vi "Measurement Coordinate Set.vi"(7 "CoordSys Type":T3(ring), 8 "error in (no error)":errorcluster, 9 "Angle (deg)":sgl, 10 "Origin":cluster{"X":sgl, "Y":sgl}, 11 "ROI Descriptor":T2 {"Contours"."Type" items=["No Selection", "Point", "Line", "Rectangle", "Oval", "Polygon", "Freehand Region", "Annulus", "Unused2", "Unused3", "Broken Line", "Freehand Line", "Rotated Rectangle"]}) -> (0 "error out":errorcluster, 2 "Coordinate System":T1 {"Measurement System"."Axis Reference" items=["Direct", "Indirect"]; "Measurement System"."Angle (deg)" format="%.2f"; "Measurement System"."Origin"."Y" format="%.2f"; "Measurement System"."Origin"."X" format="%.2f"; "Reference System"."Axis Reference" items=["Direct", "Indirect"]; "Reference System"."Angle (deg)" format="%.2f"; "Reference System"."Origin"."Y" format="%.2f"; "Reference System"."Origin"."X" format="%.2f"}, 3 "ROI Descriptor out":T2 {"Contours"."Type" items=["No Selection", "Point", "Line", "Rectangle", "Oval", "Polygon", "Freehand Region", "Annulus", "Unused2", "Unused3", "Broken Line", "Freehand Line", "Rotated Rectangle"]})   [LabVIEW 2017]
uses:
  <vilib>/vision/NI_Vision_Development_Module.lvlib
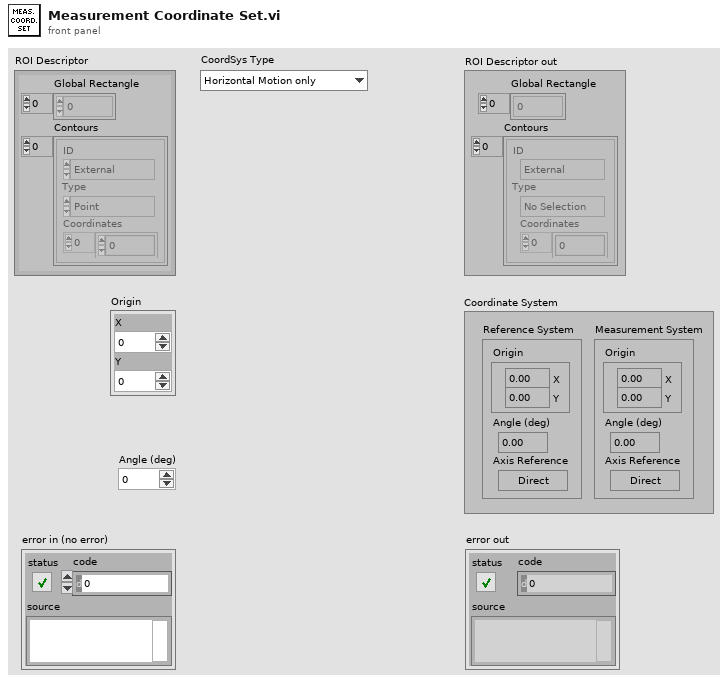
[diagram p1: front panel]
types:
  T1 = typedef "IMAQ Coordinate System" = cluster{"Reference System":cluster{"Origin":cluster{"X":sgl, "Y":sgl}, "Angle (deg)":sgl, "Axis Reference":u32}, "Measurement System":cluster{"Origin":cluster{"X":sgl, "Y":sgl}, "Angle (deg)":sgl, "Axis Reference":u32}}
  T2 = typedef "ROI Descriptor" = cluster{"Global Rectangle":i32[], "Contours":cluster{"ID":enum32{"External", "Internal"}, "Type":u32, "Coordinates":i32[]}[]}
  T3 = enum16{"Horizontal Motion only", "Vertical Motion only", "Horizontal and Vertical Motion", "Horizontal, Vertical and Angular"}
  T4 = cluster{"Origin":cluster{"X":sgl, "Y":sgl}, "Angle (deg)":sgl, "Axis Reference":u32}
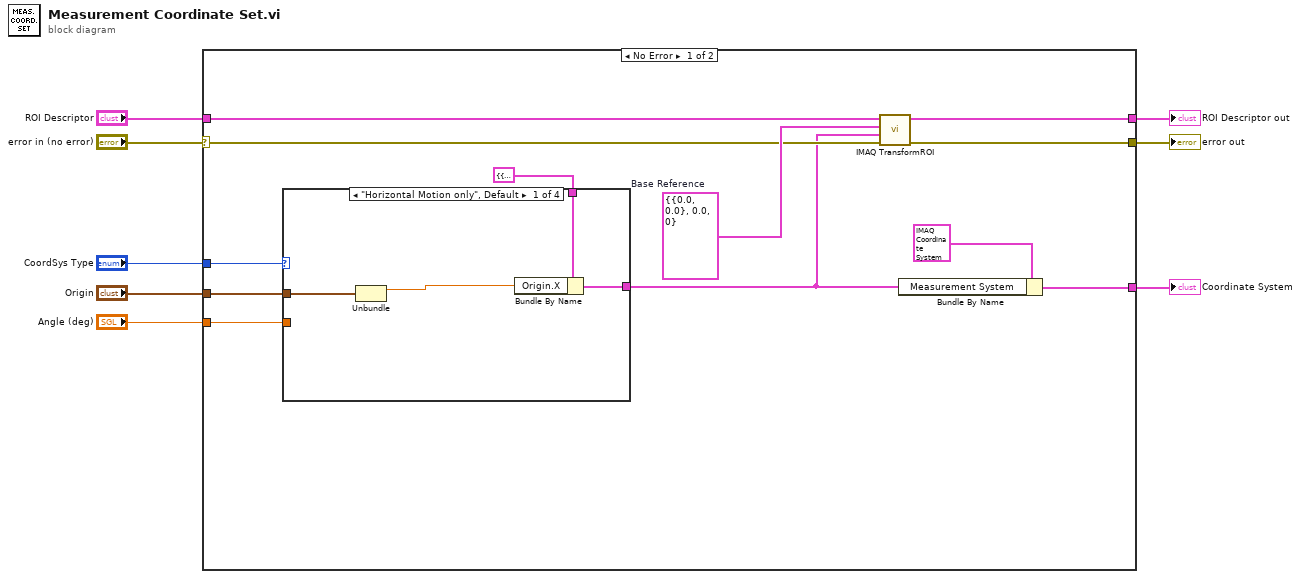
[diagram p0: block diagram]
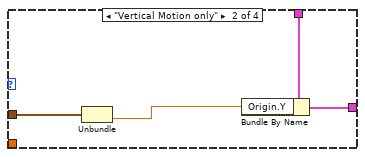
[diagram p2: hidden frame]
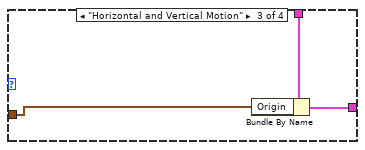
[diagram p3: hidden frame]
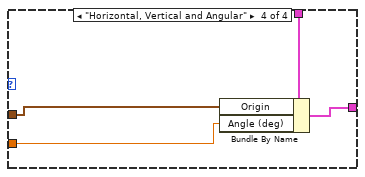
[diagram p4: hidden frame]
diagram:
  n1 = case shown="No Error" "error in (no error)" {
    selector: "error in (no error)" -> [w12 w36]
    tunnel: "CoordSys Type" -> [w20 _]
    tunnel: "Origin" -> [w18 _]
    tunnel: "Angle (deg)" -> [w17 _]
    tunnel: "ROI Descriptor" -> [w16 w37]
    tunnel: [w14 w37] -> w4
    tunnel: [w13 w36] -> w2
    tunnel: [w9 _] -> w1
    frame No Error {
      w15 = T4 {"Origin"={"X"=0.0, "Y"=0.0}, "Angle (deg)"=0.0, "Axis Reference"=0}  # Base Reference
      n2 = case shown="\"Horizontal Motion only\", Default" w20 {
        tunnel: T4 {"Origin"={"X"=0.0, "Y"=0.0}, "Angle (deg)"=0.0, "Axis Reference"=0} ("Measurement System") -> [w24 w28 w31 w35]
        tunnel: w18 -> [w22 w26 w29 w33]
        tunnel: [w23 w27 w30 w34] -> w10
        tunnel: w17 -> [_ _ _ w32]
        frame "Horizontal Motion only", Default {
          n3 = Unbundle(w22) -> ("X"=w21:sgl)  [unwired: 1 out]
          n4 = Bundle By Name(cluster=w24, "Origin.X"=w21) -> (w23:T4)
        }
        frame "Vertical Motion only" {
          n5 = Unbundle(w26) -> ("Y"=w25:sgl)  [unwired: 1 out]
          n6 = Bundle By Name(cluster=w28, "Origin.Y"=w25) -> (w27:T4)
        }
        frame "Horizontal and Vertical Motion" {
          n7 = Bundle By Name(cluster=w31, "Origin"=w29) -> (w30:T4)
        }
        frame "Horizontal, Vertical and Angular" {
          n8 = Bundle By Name(cluster=w35, "Origin"=w33, "Angle (deg)"=w32) -> (w34:T4)
        }
      }
      n9 = call "IMAQ TransformROI"("error in (no error)"=w12, "New Reference"=w10, "Base Reference"=w15, "ROI Descriptor"=w16) -> ("error out"=w13:errorcluster, "ROI Descriptor out"=w14:T2)  [unwired: 6 in]
      n10 = Bundle By Name(cluster=T1 {"Reference System"={"Origin"={"X"=0.0, "Y"=0.0}, "Angle (deg)"=0.0, "Axis Reference"=0}, "Measurement System"={"Origin"={"X"=0.0, "Y"=0.0}, "Angle (deg)"=0.0, "Axis Reference"=0}} ("Coordinate System"), "Measurement System"=w10) -> (w9:T1)
    }
    frame Error {
    }
  }
  "ROI Descriptor out" <- w4
  "error out" <- w2
  "Coordinate System" <- w1
